vi "弹窗-提示修改备注-30.vi"(0 "Enable":bool=TRUE caption="启用", 1 "信息输入":string caption="字符串", 3 "新的探头信息：":string caption="新备注", 5 "error in (no error)":errorcluster caption="错误输入（无错误）") -> (17 "新备注":string, 18 "确定":bool, 19 "error out":errorcluster caption="错误输出")   [LabVIEW 2016]
doc: "显示标准对话框，提示用户输入用户名、密码等信息。\n--------------------\n\n该Express VI配置如下:\n\n显示给用户的信息:\n该输入为: \n文本输入框: 新备注"
panel:
  in  "新的探头信息： 2":string caption="新备注"
  out "非空提示":string caption="字符串"
  out "String":string caption="字符串"
  in  "Cancel":bool caption="取消"
  in  "OK2":bool
  in  "OK1":bool
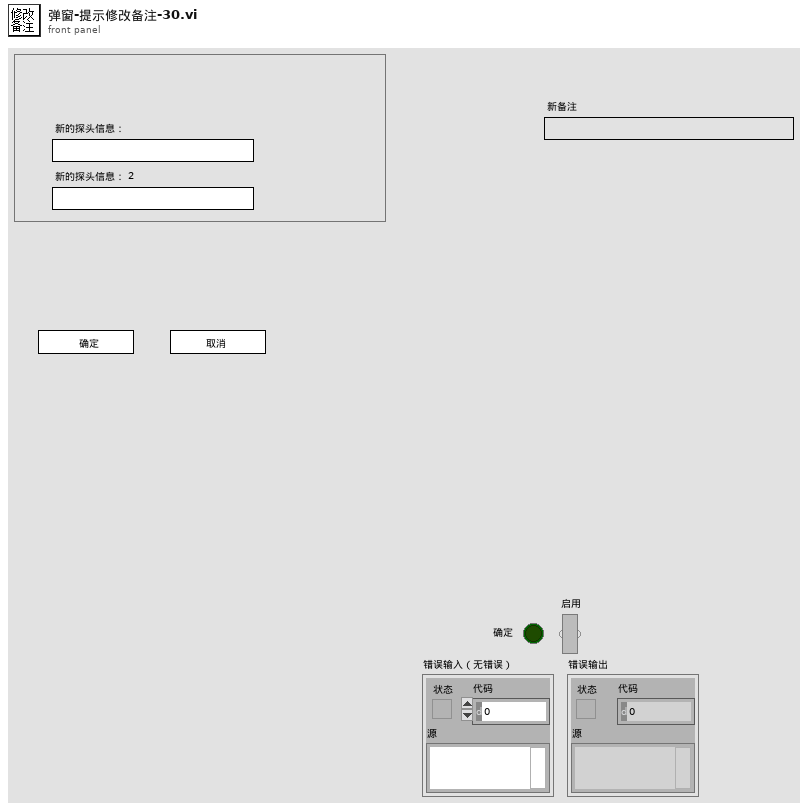
[diagram p1: front panel]
types:
  T1 = cluster{"Input Name":string, "Input Data Type":i32}[]
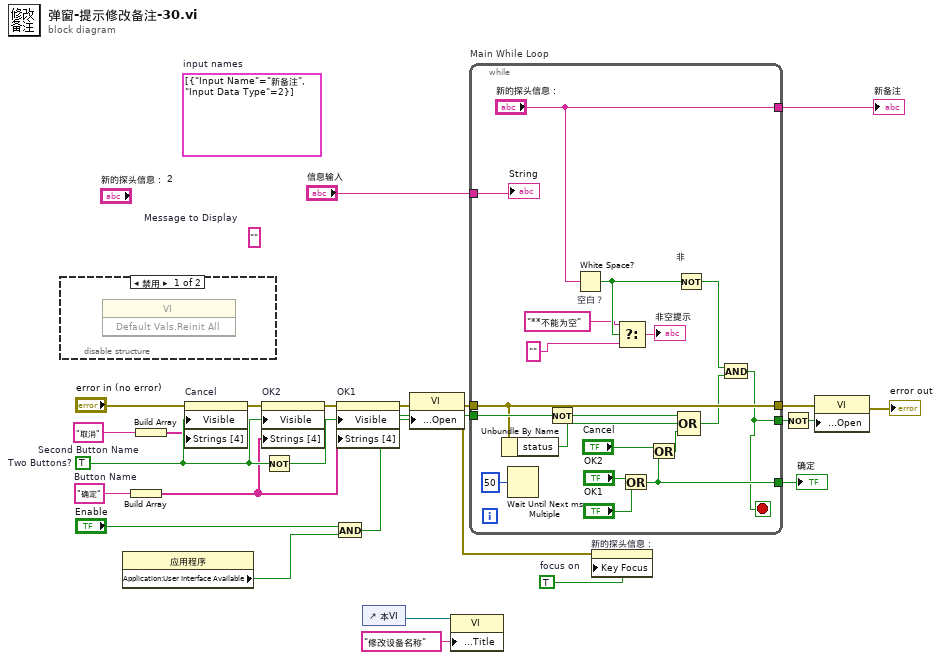
[diagram p0: block diagram]
diagram:
  w5 = TRUE  # focus on
  (unwired) T1 [{"Input Name"="新备注", "Input Data Type"=2}]  # input names
  w16 = "取消"  # Second Button Name
  w14 = "确定"  # Button Name
  (unwired) ""  # Message to Display
  w24 = TRUE  # Two Buttons?
  n1 = disable-structure shown="禁用" {
    frame Disabled {
      n2 = invoke class="VI" method="Default Vals.Reinit All"() -> ()  [unwired: 3 in, 3 out]
    }
    frame Enabled {
    }
  }
  n3 = property class="应用程序"() -> ("Application:User Interface Available"=w7:bool)  [unwired: 2 in, 2 out]
  n4 = Build Array(w14) -> (w15:string[])
  n5 = Build Array(w16) -> (w17:string[])
  n6 = property on="Cancel" class="Bool"(error in="error in (no error)", "Visible"=w24, "Strings [4]"=w17) -> (error out=w21:errorcluster)  [unwired: 1 in, 1 out]
  n7 = property on="OK2" class="Bool"(error in=w21, "Visible"=w24, "Strings [4]"=w15) -> (error out=w20:errorcluster)  [unwired: 1 in, 1 out]
  n8 = Not(x=w24) -> (.not. x?=w22:bool)
  n9 = And(x="Enable", y=w7) -> (x .and. y?=w8:bool)
  n10 = property on="OK1" class="Bool"(error in=w20, "Visible"=w22, "Strings [4]"=w15) -> (error out=w13:errorcluster)  [unwired: 1 in, 1 out]
  n11 = control-ref of="本VI"() -> (w3:refnum<vi>)
  n12 = property class="VI"(error in=w13, "Front Panel Window:Open"=w8) -> (error out=w12:errorcluster)  [unwired: 1 in, 1 out]
  n13 = property class="VI"(reference=w3, "Front Panel.Title"="修改设备名称" ("前面板窗口:标题")) -> ()  [unwired: 1 in, 2 out]
  n14 = while "Main While Loop" {
    tunnel: [w40] -> w23
    tunnel: w8 -> [w38]
    tunnel: [w29] -> w18
    tunnel: w12 -> [w36]
    tunnel: [w36] -> w10
    tunnel: ["新的探头信息："] -> w6
    tunnel: "信息输入" -> [w33]
    stop <- w29 stop-if-true
    n15 = Unbundle By Name(w36) -> ("status"=w34:bool)
    n16 = Wait Until Next ms Multiple(millisecond multiple=u32 50) -> ()  [unwired: 1 out]
    n17 = Not(x=w38) -> (.not. x?=w37:bool)
    n18 = White Space? "空白？"(1:"新的探头信息：") -> (0:w27:bool)
    n19 = Select(t="**不能为空", s=w27, f="") -> (s? t:f=→"非空提示":string)
    n20 = Or(x="OK2", y="OK1") -> (x .or. y?=w40:bool)
    n21 = Or(x="Cancel", y=w40) -> (x .or. y?=w35:bool)
    n22 = Not "非"(x=w27) -> (.not. x?=w30:bool)
    n23 = Compound Arithmetic op=OR(w37, w34, w35) -> (w31:bool)
    n24 = And(x=w30, y=w31) -> (x .and. y?=w29:bool)
    "String" <- w33
  }
  "确定" <- w23
  "新备注" <- w6
  n25 = property on="新的探头信息：" class="Str"(error in=w12, "Key Focus"=w5) -> ()  [unwired: 1 in, 2 out]
  n26 = Not(x=w18) -> (.not. x?=w19:bool)
  n27 = property class="VI"(error in=w10, "Front Panel Window:Open"=w19) -> (error out=→"error out":errorcluster)  [unwired: 1 in, 1 out]
